vi "CreateCore.vi"(5 "Backends":T1, 7 "Target":T2, 8 "error in (no error)":errorcluster, 9 "Model Properties":T3, 10 "Config File":path, 11 "Model File":path) -> (0 "error out":errorcluster, 3 "DNN Detection Model":refnum<class "DNN Detection Model.lvclass">)   [LabVIEW 2020, in "feature_detection.lvlib" / "DNN Detection Model.lvclass"]
uses:
  DNN Detection Model.lvclass
  Model Parameters.ctl
  common/Image Size (Integer).ctl
  common/Object Point (Float).ctl
  Targets.ctl
  Backends.ctl
  DNN Detection Model.lvclass/DNN Detection Model.ctl
  common/common.lvlib
  common/bin/gartoolkit_dnn_32-1.dll
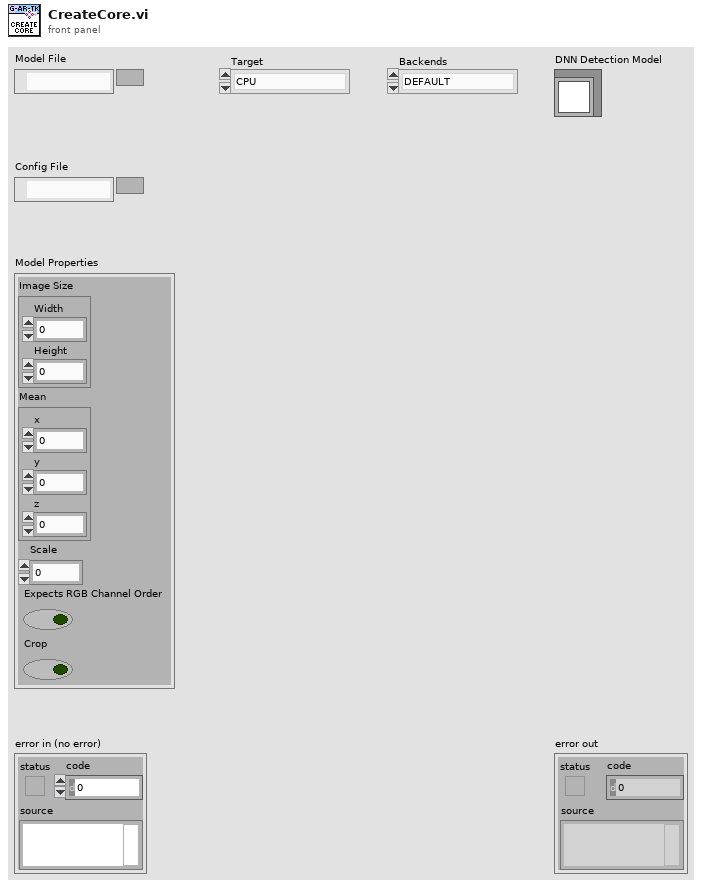
[diagram p1: front panel]
types:
  T1 = typedef "feature_detection.lvlib/DNN Detection Model.lvclass/Backends.ctl" = enum8{"DEFAULT", "HALIDE", "INFERENCE_ENGINE", "OPENCV", "VKCOM", "CUDA", "WEBNN", "TIMVX", "CANN"}
  T2 = typedef "feature_detection.lvlib/DNN Detection Model.lvclass/Targets.ctl" = enum16{"CPU", "OPENCL", "OPENCL_FP16", "MYRIAD", "VULKAN", "FPGA", "CUDA", "CUDA_FP16", "HDDL", "NPU", "CPU_FP16"}
  T3 = typedef "feature_detection.lvlib/DNN Detection Model.lvclass/Model Parameters.ctl" = cluster{"Image Size":T4, "Mean":T5, "Scale":dbl, "Expects RGB Channel Order":bool, "Crop":bool}
  T4 = typedef "common.lvlib/Image Size (Integer).ctl" = cluster{"Width":u16, "Height":u16}
  T5 = typedef "common.lvlib/Object Point (Float).ctl" = cluster{"x":dbl, "y":dbl, "z":dbl}
  T6 = cluster{"Path String":string, "Path String":string, "Image Size":T4, "Mean":T5, "Scale":dbl, "Expects RGB Channel Order":bool, "Crop":bool}
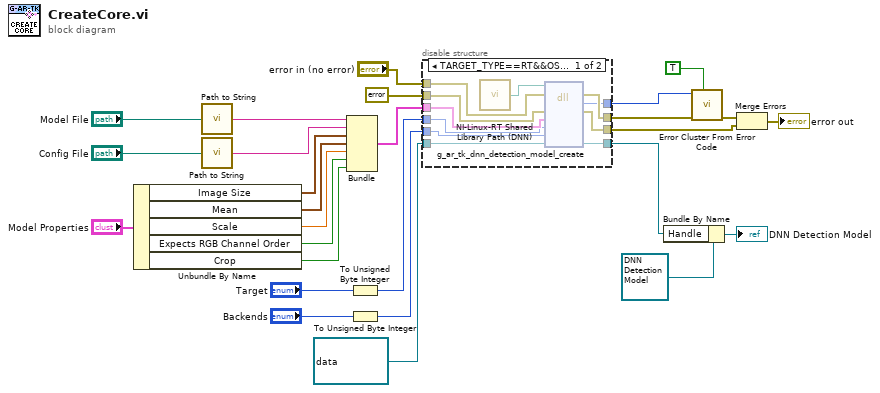
[diagram p0: block diagram]
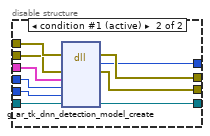
[diagram p2: hidden frame]
diagram:
  n1 = Unbundle By Name("Model Properties") -> ("Image Size"=w16:T4, "Mean"=w17:T5, "Scale"=w18:dbl, "Expects RGB Channel Order"=w19:bool, "Crop"=w11:bool)
  n2 = call "Path to String.vi"("Path"="Model File") -> ("Path String"=w15:string)
  n3 = call "Path to String.vi"("Path"="Config File") -> ("Path String"=w14:string)
  n4 = Bundle("Path String"=w15, "Path String"=w14, "Image Size"=w16, "Mean"=w17, "Scale"=w18, "Expects RGB Channel Order"=w19, "Crop"=w11) -> (w13:T6)  [unwired: 1 in]
  n5 = To Unsigned Byte Integer(number="Target") -> (unsigned 8bit integer=w9:u8)
  n6 = To Unsigned Byte Integer(number="Backends") -> (unsigned 8bit integer=w7:u8)
  n7 = disable-structure "Conditional Disable Structure" shown="TARGET_TYPE==RT&&OS==Linux" {
    disable-tunnel: "error in (no error)" -> [w38 w48]
    disable-tunnel: errorcluster {"status"=FALSE, "code"=0, "source"=""} ("error constant") -> [w37 w47]
    disable-tunnel: refnum<data-value> refnum ("EDVR") -> [w33 w46]
    disable-tunnel: [w31 w45] -> w24
    disable-tunnel: [w29 w44] -> w23
    disable-tunnel: [w28 w43] -> w22
    disable-tunnel: [w30 w42] -> w21
    disable-tunnel: w13 -> [w36 w41]
    disable-tunnel: w9 -> [w35 w40]
    disable-tunnel: w7 -> [w34 w39]
    frame condition #0 {
      n8 = call "NI-Linux-RT Shared Library Path (DNN).vi"() -> ("Path"=w32:path)
      n9 = dll-call lib="?" fn="g_ar_tk_dnn_detection_model_create" ("g_ar_toolkit.*.*:g_ar_tk_capture_context_create")(path in=w32, error in=w38, "error_cluster"=w37, "model"=w36, "Target"=w35, "Backend"=w34, "EDVR"=w33) -> (error out=w31:errorcluster, "return type"=w29:i32, "error_cluster"=w30:errorcluster, "EDVR"=w28:refnum<data-value>)  [unwired: 4 in, 1 out]
    }
    frame condition #1 (active) {
      n10 = dll-call lib="C:/serenial/lib/g-augmented-reality-toolkit/LabVIEW/common/bin/gartoolkit_dnn_*-1.*" fn="g_ar_tk_dnn_detection_model_create" ("g_ar_toolkit.*.*:g_ar_tk_capture_context_create")(error in=w48, "error_cluster"=w47, "model"=w41, "Target"=w40, "Backend"=w39, "EDVR"=w46) -> (error out=w45:errorcluster, "return type"=w44:i32, "error_cluster"=w42:errorcluster, "EDVR"=w43:refnum<data-value>)  [unwired: 5 in, 1 out]
    }
  }
  n11 = Bundle By Name(cluster=refnum<class "DNN Detection Model.lvclass"> refnum ("feature_detection.lvlib:DNN Detection Model.lvclass"), "Handle"=w22) -> (→"DNN Detection Model":refnum<class "DNN Detection Model.lvclass">)
  n12 = call <vilib>:"Error Cluster From Error Code.vi"("show call chain? (False)"=TRUE, "error in (no error)"=w24, "error code (0)"=w23) -> ("error out"=w27:errorcluster)  [unwired: 6 in]
  n13 = Merge Errors(w27, w21) -> (→"error out":errorcluster)
